vi "Labview8_3.vi"(1 "Input 4":dbl, 2 "Input 3":dbl, 3 "Input 2":dbl, 4 "Input 1":dbl) -> (0 "Output 5":dbl)   [LabVIEW 2016]
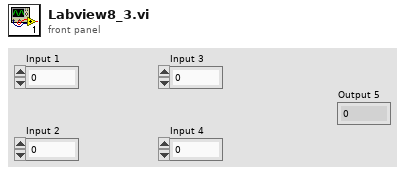
[diagram p1: front panel]
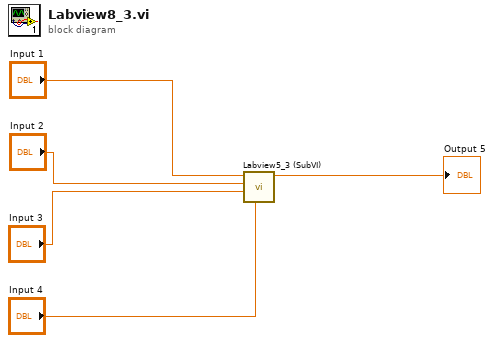
[diagram p0: block diagram]
diagram:
  n1 = call "Labview5_3 (SubVI).vi"("Input 4"="Input 4", "Input 3"="Input 3", "Input in"="Input 2", "Input 1"="Input 1") -> ("Numeric"=→"Output 5":dbl)  [unwired: 7 in]
